vi "Set Speed.vi"(8 "error in (no error)":errorcluster, 10 "Speed (%)":dbl, 11 "Ismatech 3 Channel Settings In":T1={"VISA resource name"="", "Pump Number"=1, "Channel Number"=0, "Simulated?"=TRUE, "Reverse?"=FALSE} {"Channel Number" min=0 max=3; "Pump Number" min=1 max=9}) -> (0 "error out":errorcluster, 1 "Connection Error":bool, 2 "3 Fails":bool, 3 "Ismatech 3 Channel Settings Out":T1={"VISA resource name"="", "Pump Number"=1, "Channel Number"=0, "Simulated?"=TRUE, "Reverse?"=FALSE} {"Channel Number" min=0 max=3; "Pump Number" min=1 max=9})   [LabVIEW 2018, in "Ismatec 4308.lvlib"]
uses:
  Ismatec 4308.lvlib
  Ismatec 4083.ctl
  support/Support Library.lvlib
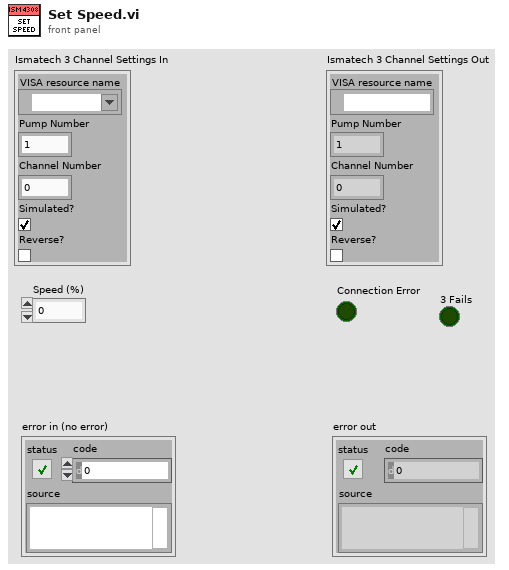
[diagram p1: front panel]
types:
  T1 = typedef "Ismatec 4308.lvlib/Ismatec 4083.ctl" = cluster{"VISA resource name":refnum<visa-resource-name>, "Pump Number":i16, "Channel Number":i16, "Simulated?":bool, "Reverse?":bool}
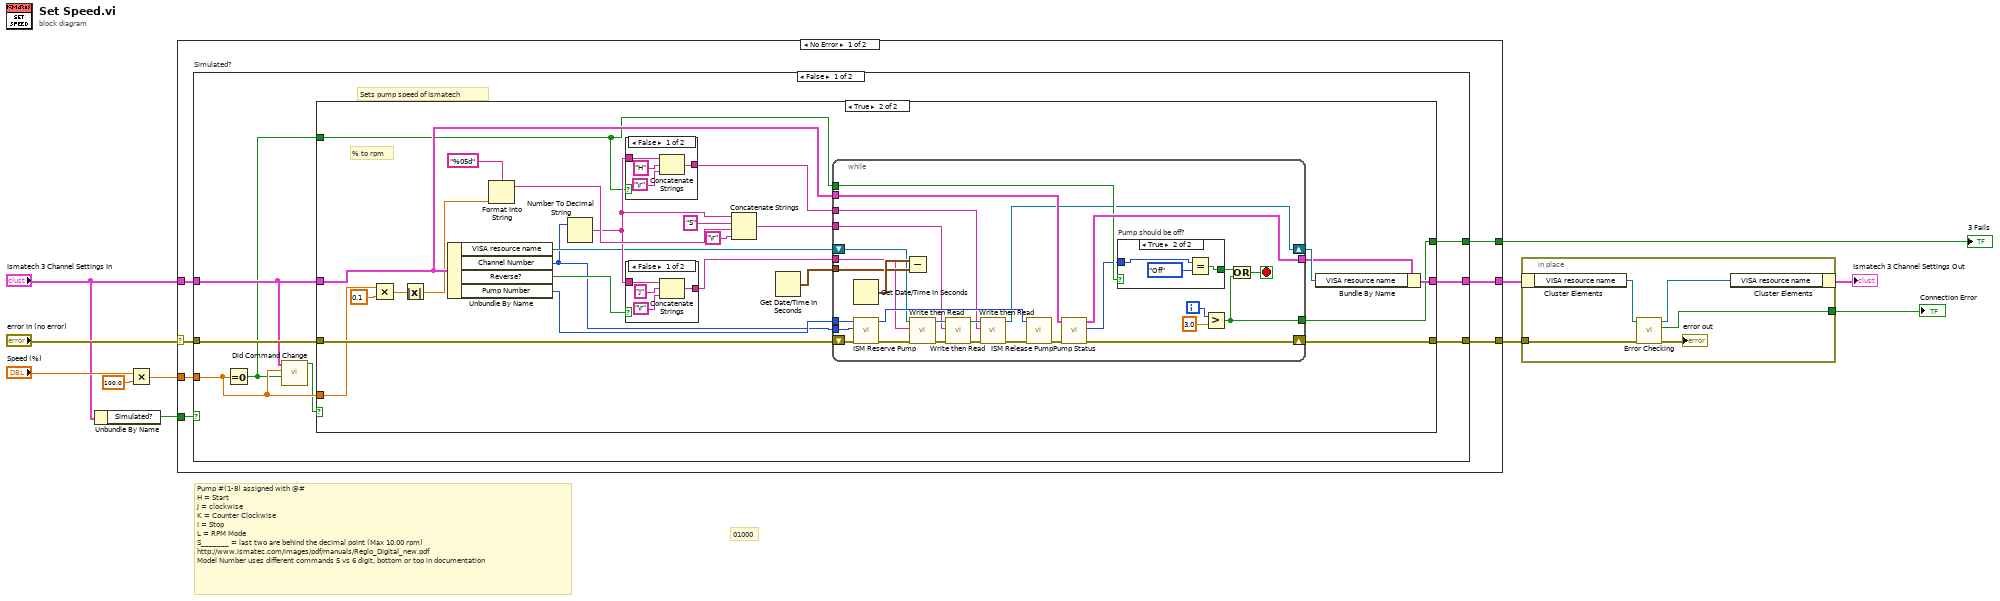
[diagram p0: block diagram]
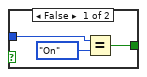
[diagram p3: hidden frame]
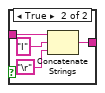
[diagram p4: hidden frame]
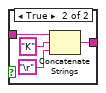
[diagram p5: hidden frame]
diagram:
  # "01000"
  # "Pump #(1-8) assigned with @#\nH = Start\nJ = clockwise\nK = Counter Clockwise\nI = Stop\nL = RPM Mode\nS_______ = last two are behind the decimal point (Max 10.00 rpm)\nhttp://www.ismatec.com/images/pdf/manuals/Reglo_Digital_new.pdf\nModel Number uses different commands 5 vs 6 digit, bottom or top in documentation"
  n1 = Unbundle By Name("Ismatech 3 Channel Settings In") -> ("Simulated?"=w10:bool)
  n2 = Multiply(x="Speed (%)", y=100.0) -> (x*y=w6:dbl)
  n3 = case shown="No Error" "error in (no error)" {
    selector: "error in (no error)" -> [w16 w107]
    tunnel: [w14 w106] -> w4
    tunnel: [w13 w107] -> w9
    tunnel: w6 -> [w15 _]
    tunnel: "Ismatech 3 Channel Settings In" -> [w18 w106]
    tunnel: w10 -> [w17 _]
    tunnel: [w12 _] -> w1
    frame No Error {
      n4 = case "Simulated?" shown="False" w17 {
        tunnel: w15 -> [w22 _]
        tunnel: w18 -> [w23 w105]
        tunnel: [w26 w105] -> w14
        tunnel: w16 -> [w25 w104]
        tunnel: [w24 w104] -> w13
        tunnel: [w19 _] -> w12
        frame False {
          # "Sets pump speed of Ismatech"
          n5 = Equal To 0?(x=w22) -> (x = 0?=w21:bool)
          n6 = call "Did Command Change.vi"("Paused"=w21, "Numeric"=w22, "Ismatech 3 Channel Settings In"=w23) -> ("Change"=w20:bool)  [unwired: 8 in]
          n7 = case shown="True" w20 {
            tunnel: [w28 w53] -> w26
            tunnel: w25 -> [w27 w47]
            tunnel: [w27 w42] -> w24
            tunnel: w22 -> [_ w35]
            tunnel: w23 -> [w28 w34]
            tunnel: w21 -> [_ w32]
            tunnel: [_ w30] -> w19
            frame False {
            }
            frame True {
              # "% to rpm"
              n8 = Multiply(x=w35, y=0.1) -> (x*y=w37:dbl)
              n9 = Absolute Value(x=w37) -> (abs(x)=w33:dbl)
              n10 = Unbundle By Name(w34) -> ("VISA resource name"=w36:refnum<visa-resource-name>, "Channel Number"=w29:i16, "Reverse?"=w43:bool, "Pump Number"=w31:i16)
              n11 = Format Into String(format string="%05d", w33) -> (resulting string=w50:string)  [unwired: 2 in, 1 out]
              n12 = Number To Decimal String(number=w29) -> (decimal integer string=w40:string)  [unwired: 1 in]
              n13 = case shown="False" w32 {
                tunnel: [w89 w92] -> w44
                tunnel: w40 -> [w88 w93]
                frame False {
                  n14 = Concatenate Strings(w88, "H", "\r") -> (w89:string)
                }
                frame True {
                  n15 = Concatenate Strings(w93, "I", "\r") -> (w92:string)
                }
              }
              n16 = case shown="False" w43 {
                tunnel: w40 -> [w98 w103]
                tunnel: [w97 w101] -> w46
                frame False {
                  n17 = Concatenate Strings(w98, "J" ("string"), "\r") -> (w97:string)
                }
                frame True {
                  n18 = Concatenate Strings(w103, "K" ("string"), "\r") -> (w101:string)
                }
              }
              n19 = Concatenate Strings(w40, "S" ("string"), w50, "\r") -> (w45:string)
              n20 = Get Date/Time In Seconds() -> (seconds since 1Jan1904=w38:timestamp)
              n21 = while {
                tunnel: w46 -> [w64]
                tunnel: w45 -> [w61]
                tunnel: w44 -> [w58]
                shift-right: [w81] -> w42
                shift-left: w47 -> [w71]
                shift-right: [w55] -> w41
                shift-left: w36 -> [w65]
                tunnel: w32 -> [w77]
                tunnel: w34 -> [w79]
                tunnel: [w78] -> w39
                tunnel: w38 -> [w72]
                tunnel: w31 -> [w70]
                tunnel: [w68] -> w30
                tunnel: w29 -> [w54]
                i -> [w66]
                stop <- w74 stop-if-true
                n22 = Get Date/Time In Seconds() -> (seconds since 1Jan1904=w73:timestamp)
                n23 = call "ISM Reserve Pump.vi"("error in (no error)"=w71, "ISM Channel # In"=w54, "ISM Pump # In"=w70) -> ("error out"=w63:errorcluster, "ISM Pump # Out"=w69:i32)  [unwired: 7 in]
                n24 = Subtract(x=w73, y=w72) -> ()  [unwired: 1 out]
                n25 = call "Write then Read.vi"("error in"=w63, "write buffer"=w64, "VISA resource name in"=w65) -> ("error out"=w60:errorcluster, "VISA resource name out"=w62:refnum<visa-resource-name>)  [unwired: 6 in, 1 out]
                n26 = call "Write then Read.vi"("error in"=w60, "write buffer"=w61, "VISA resource name in"=w62) -> ("error out"=w57:errorcluster, "VISA resource name out"=w59:refnum<visa-resource-name>)  [unwired: 6 in, 1 out]
                n27 = call "Write then Read.vi"("error in"=w57, "write buffer"=w58, "VISA resource name in"=w59) -> ("error out"=w56:errorcluster, "VISA resource name out"=w55:refnum<visa-resource-name>)  [unwired: 6 in, 1 out]
                n28 = call "ISM Release Pump.vi"("error in (no error)"=w56, "Pump Number In"=w69) -> ("error out"=w80:errorcluster)  [unwired: 8 in, 1 out]
                n29 = call "Pump Status.vi"("error in (no error)"=w80, "Ismatech 3 Channel Settings In"=w79) -> ("error out"=w81:errorcluster, "Pump On?"=w67:enum16{"Off", "On", "Not Initialized"}, "Ismatech 3 Channel Settings Out"=w78:T1)  [unwired: 5 in, 2 out]
                n30 = case "Pump should be off?" shown="True" w77 {
                  tunnel: [w82 w85] -> w75
                  tunnel: w67 -> [w83 w86]
                  frame False {
                    n31 = Equal?(x=w83, y=enum16{"Off", "On", "Not Initialized"}."On") -> (x = y?=w82:bool)
                  }
                  frame True {
                    n32 = Equal?(x=w86, y=enum16{"Off", "On", "Not Initialized"}."Off") -> (x = y?=w85:bool)
                  }
                }
                n33 = Greater?(x=w66, y=3.0) -> (0:w68:bool)
                n34 = Or(x=w75, y=w68) -> (x .or. y?=w74:bool)
              }
              n35 = Bundle By Name(cluster=w39, "VISA resource name"=w41) -> (w53:T1)
            }
          }
        }
        frame True {
        }
      }
    }
    frame Error {
    }
  }
  "3 Fails" <- w1
  n36 = in-place {
    in-place-border: w9 -> [w112]
    in-place-border: [w110] -> w5
    n37 = in-place-cluster #1(w4) -> ("VISA resource name"=w109:refnum<visa-resource-name>)
    n38 = call "Error Checking.vi"("error in (no error)"=w112, "VISA resource name"=w109) -> ("error out"=→"error out":errorcluster, "Connection Error"=w110:bool, "VISA resource name"=w108:refnum<visa-resource-name>)  [unwired: 7 in]
    n39 = in-place-cluster #1("VISA resource name"=w108) -> (→"Ismatech 3 Channel Settings Out":T1)
  }
  "Connection Error" <- w5
